vi "Solenoid Bank.vi"(0 "VISA session":refnum<visa-resource-name>="MW100", 1 "Semiphore":T1, 2 "Valve Bank":u16(ring) items=["A", "B", "C", "D"], 5 "Drain Valve":enum8{"OPEN", "CLOSE"}(ring)=enum."CLOSE", 7 "Output Valve":enum8{"CLOSE", "OPEN"}(ring)=enum."OPEN", 9 "Input Valve":enum8{"OPEN", "CLOSE"}(ring)=enum."CLOSE", 11 "Error In":errorcluster) -> (4 "dup VISA session":refnum<visa-resource-name>, 15 "Error Out":errorcluster)   [LabVIEW 2012]
uses:
  ChannelSettings.ctl
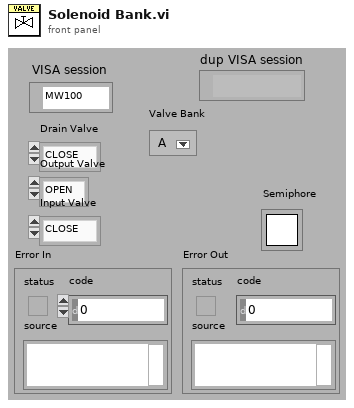
[diagram p1: front panel]
types:
  T1 = typedef "Semaphore RefNum" = refnum<k1>
  T2 = typedef "ChannelSettings.ctl" = u32
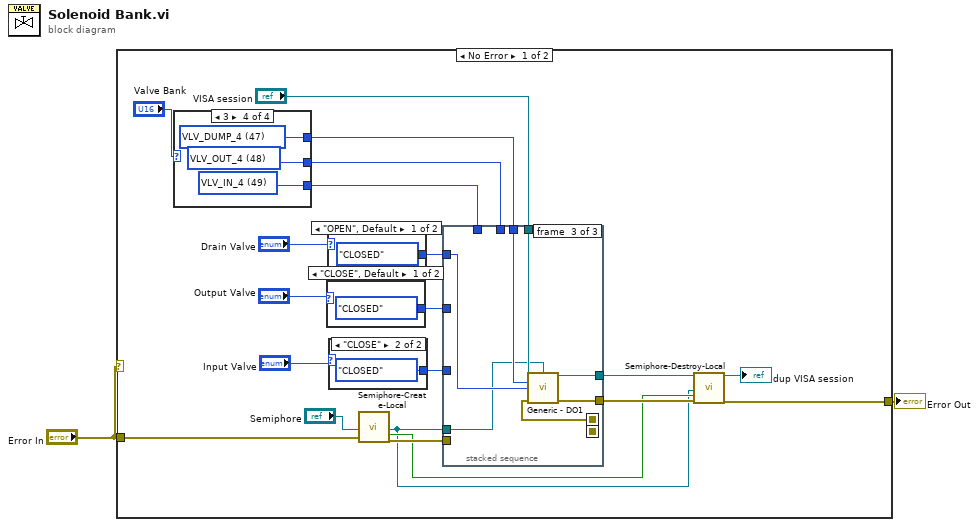
[diagram p0: block diagram]
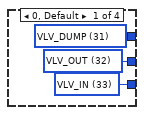
[diagram p2: hidden frame]
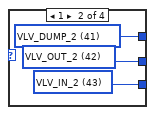
[diagram p3: hidden frame]
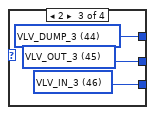
[diagram p4: hidden frame]
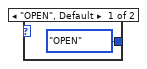
[diagram p5: hidden frame]
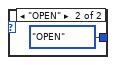
[diagram p6: hidden frame]
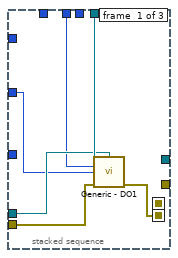
[diagram p7: hidden frame]
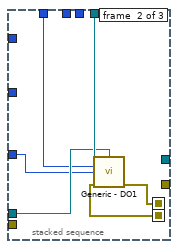
[diagram p8: hidden frame]
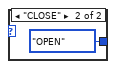
[diagram p9: hidden frame]
diagram:
  n1 = case shown="No Error" "Error In" {
    tunnel: "Error In" -> [w15 w59]
    tunnel: [w12 w59] -> w1
    frame No Error {
      n2 = case shown="3" "Valve Bank" {
        tunnel: [w24 w27 w30 w33] -> w17
        tunnel: [w23 w26 w29 w32] -> w5
        tunnel: [w22 w25 w28 w31] -> w4
        frame 0, Default {
          w22 = T2 33 items=["4-20_OUT", "Pres_HI1", "Pres_HI2", "Pres_LOW", "Pres_PIN", "HEATER_TOP", "HEATER_BOT", "T_Shell", "FLOWMETER", "WATT_SENSE", "WH_TICK", "Tc_1", "Tc_2", "Tc_3", "Tc_4", "Tc_5", "Tc_6", "Tc_down", "T_Shell_2", "T_Shell_3", "T_Shell_4", "RTD_IN", "RTD_OUT", "RTD_AMB", "INTF_TEMPFLO", "INTF_READY", "INTF_START", "INTF_STOP", "DRM_LOW", "DRM_HIGH", "PWR_MAIN", "VLV_DUMP", "VLV_OUT", "VLV_IN", "WATT_HOURS", "FLOW(SAMPLE)", "GALLONS", "FLOW(GPM)"] ("Channel_Enum")
          w23 = T2 32 items=["4-20_OUT", "Pres_HI1", "Pres_HI2", "Pres_LOW", "Pres_PIN", "HEATER_TOP", "HEATER_BOT", "T_Shell", "FLOWMETER", "WATT_SENSE", "WH_TICK", "Tc_1", "Tc_2", "Tc_3", "Tc_4", "Tc_5", "Tc_6", "Tc_down", "T_Shell_2", "T_Shell_3", "T_Shell_4", "RTD_IN", "RTD_OUT", "RTD_AMB", "INTF_TEMPFLO", "INTF_READY", "INTF_START", "INTF_STOP", "DRM_LOW", "DRM_HIGH", "PWR_MAIN", "VLV_DUMP", "VLV_OUT", "VLV_IN", "WATT_HOURS", "FLOW(SAMPLE)", "GALLONS", "FLOW(GPM)"] ("Channel_Enum")
          w24 = T2 31 items=["4-20_OUT", "Pres_HI1", "Pres_HI2", "Pres_LOW", "Pres_PIN", "HEATER_TOP", "HEATER_BOT", "T_Shell", "FLOWMETER", "WATT_SENSE", "WH_TICK", "Tc_1", "Tc_2", "Tc_3", "Tc_4", "Tc_5", "Tc_6", "Tc_down", "T_Shell_2", "T_Shell_3", "T_Shell_4", "RTD_IN", "RTD_OUT", "RTD_AMB", "INTF_TEMPFLO", "INTF_READY", "INTF_START", "INTF_STOP", "DRM_LOW", "DRM_HIGH", "PWR_MAIN", "VLV_DUMP", "VLV_OUT", "VLV_IN", "WATT_HOURS", "FLOW(SAMPLE)", "GALLONS", "FLOW(GPM)"] ("Channel_Enum")
        }
        frame 1 {
          w25 = T2 43 items=["4-20_OUT", "Pres_HI1", "Pres_HI2", "Pres_LOW", "Pres_PIN", "HEATER_TOP", "HEATER_BOT", "T_Shell", "FLOWMETER", "WATT_SENSE", "WH_TICK", "Tc_1", "Tc_2", "Tc_3", "Tc_4", "Tc_5", "Tc_6", "Tc_down", "T_Shell_2", "T_Shell_3", "T_Shell_4", "RTD_IN", "RTD_OUT", "RTD_AMB", "INTF_TEMPFLO", "INTF_READY", "INTF_START", "INTF_STOP", "DRM_LOW", "DRM_HIGH", "PWR_MAIN", "VLV_DUMP", "VLV_OUT", "VLV_IN", "WATT_HOURS", "FLOW(SAMPLE)", "GALLONS", "FLOW(GPM)", "FLOW_CALC_GAIN", "FLOW_CALC_OFFSET", "FLOW_CALC_THRESHOLD", "VLV_DUMP_2", "VLV_OUT_2", "VLV_IN_2", "VLV_DUMP_3", "VLV_OUT_3", "VLV_IN_3", "VLV_DUMP_4", "VLV_OUT_4", "VLV_IN_4"] ("Channel_Enum")
          w26 = T2 42 items=["4-20_OUT", "Pres_HI1", "Pres_HI2", "Pres_LOW", "Pres_PIN", "HEATER_TOP", "HEATER_BOT", "T_Shell", "FLOWMETER", "WATT_SENSE", "WH_TICK", "Tc_1", "Tc_2", "Tc_3", "Tc_4", "Tc_5", "Tc_6", "Tc_down", "T_Shell_2", "T_Shell_3", "T_Shell_4", "RTD_IN", "RTD_OUT", "RTD_AMB", "INTF_TEMPFLO", "INTF_READY", "INTF_START", "INTF_STOP", "DRM_LOW", "DRM_HIGH", "PWR_MAIN", "VLV_DUMP", "VLV_OUT", "VLV_IN", "WATT_HOURS", "FLOW(SAMPLE)", "GALLONS", "FLOW(GPM)", "FLOW_CALC_GAIN", "FLOW_CALC_OFFSET", "FLOW_CALC_THRESHOLD", "VLV_DUMP_2", "VLV_OUT_2", "VLV_IN_2", "VLV_DUMP_3", "VLV_OUT_3", "VLV_IN_3", "VLV_DUMP_4", "VLV_OUT_4", "VLV_IN_4"] ("Channel_Enum")
          w27 = T2 41 items=["4-20_OUT", "Pres_HI1", "Pres_HI2", "Pres_LOW", "Pres_PIN", "HEATER_TOP", "HEATER_BOT", "T_Shell", "FLOWMETER", "WATT_SENSE", "WH_TICK", "Tc_1", "Tc_2", "Tc_3", "Tc_4", "Tc_5", "Tc_6", "Tc_down", "T_Shell_2", "T_Shell_3", "T_Shell_4", "RTD_IN", "RTD_OUT", "RTD_AMB", "INTF_TEMPFLO", "INTF_READY", "INTF_START", "INTF_STOP", "DRM_LOW", "DRM_HIGH", "PWR_MAIN", "VLV_DUMP", "VLV_OUT", "VLV_IN", "WATT_HOURS", "FLOW(SAMPLE)", "GALLONS", "FLOW(GPM)", "FLOW_CALC_GAIN", "FLOW_CALC_OFFSET", "FLOW_CALC_THRESHOLD", "VLV_DUMP_2", "VLV_OUT_2", "VLV_IN_2", "VLV_DUMP_3", "VLV_OUT_3", "VLV_IN_3", "VLV_DUMP_4", "VLV_OUT_4", "VLV_IN_4"] ("Channel_Enum")
        }
        frame 2 {
          w28 = T2 46 items=["4-20_OUT", "Pres_HI1", "Pres_HI2", "Pres_LOW", "Pres_PIN", "HEATER_TOP", "HEATER_BOT", "T_Shell", "FLOWMETER", "WATT_SENSE", "WH_TICK", "Tc_1", "Tc_2", "Tc_3", "Tc_4", "Tc_5", "Tc_6", "Tc_down", "T_Shell_2", "T_Shell_3", "T_Shell_4", "RTD_IN", "RTD_OUT", "RTD_AMB", "INTF_TEMPFLO", "INTF_READY", "INTF_START", "INTF_STOP", "DRM_LOW", "DRM_HIGH", "PWR_MAIN", "VLV_DUMP", "VLV_OUT", "VLV_IN", "WATT_HOURS", "FLOW(SAMPLE)", "GALLONS", "FLOW(GPM)", "FLOW_CALC_GAIN", "FLOW_CALC_OFFSET", "FLOW_CALC_THRESHOLD", "VLV_DUMP_2", "VLV_OUT_2", "VLV_IN_2", "VLV_DUMP_3", "VLV_OUT_3", "VLV_IN_3", "VLV_DUMP_4", "VLV_OUT_4", "VLV_IN_4"] ("Channel_Enum")
          w29 = T2 45 items=["4-20_OUT", "Pres_HI1", "Pres_HI2", "Pres_LOW", "Pres_PIN", "HEATER_TOP", "HEATER_BOT", "T_Shell", "FLOWMETER", "WATT_SENSE", "WH_TICK", "Tc_1", "Tc_2", "Tc_3", "Tc_4", "Tc_5", "Tc_6", "Tc_down", "T_Shell_2", "T_Shell_3", "T_Shell_4", "RTD_IN", "RTD_OUT", "RTD_AMB", "INTF_TEMPFLO", "INTF_READY", "INTF_START", "INTF_STOP", "DRM_LOW", "DRM_HIGH", "PWR_MAIN", "VLV_DUMP", "VLV_OUT", "VLV_IN", "WATT_HOURS", "FLOW(SAMPLE)", "GALLONS", "FLOW(GPM)", "FLOW_CALC_GAIN", "FLOW_CALC_OFFSET", "FLOW_CALC_THRESHOLD", "VLV_DUMP_2", "VLV_OUT_2", "VLV_IN_2", "VLV_DUMP_3", "VLV_OUT_3", "VLV_IN_3", "VLV_DUMP_4", "VLV_OUT_4", "VLV_IN_4"] ("Channel_Enum")
          w30 = T2 44 items=["4-20_OUT", "Pres_HI1", "Pres_HI2", "Pres_LOW", "Pres_PIN", "HEATER_TOP", "HEATER_BOT", "T_Shell", "FLOWMETER", "WATT_SENSE", "WH_TICK", "Tc_1", "Tc_2", "Tc_3", "Tc_4", "Tc_5", "Tc_6", "Tc_down", "T_Shell_2", "T_Shell_3", "T_Shell_4", "RTD_IN", "RTD_OUT", "RTD_AMB", "INTF_TEMPFLO", "INTF_READY", "INTF_START", "INTF_STOP", "DRM_LOW", "DRM_HIGH", "PWR_MAIN", "VLV_DUMP", "VLV_OUT", "VLV_IN", "WATT_HOURS", "FLOW(SAMPLE)", "GALLONS", "FLOW(GPM)", "FLOW_CALC_GAIN", "FLOW_CALC_OFFSET", "FLOW_CALC_THRESHOLD", "VLV_DUMP_2", "VLV_OUT_2", "VLV_IN_2", "VLV_DUMP_3", "VLV_OUT_3", "VLV_IN_3", "VLV_DUMP_4", "VLV_OUT_4", "VLV_IN_4"] ("Channel_Enum")
        }
        frame 3 {
          w31 = T2 49 items=["4-20_OUT", "Pres_HI1", "Pres_HI2", "Pres_LOW", "Pres_PIN", "HEATER_TOP", "HEATER_BOT", "T_Shell", "FLOWMETER", "WATT_SENSE", "WH_TICK", "Tc_1", "Tc_2", "Tc_3", "Tc_4", "Tc_5", "Tc_6", "Tc_down", "T_Shell_2", "T_Shell_3", "T_Shell_4", "RTD_IN", "RTD_OUT", "RTD_AMB", "INTF_TEMPFLO", "INTF_READY", "INTF_START", "INTF_STOP", "DRM_LOW", "DRM_HIGH", "PWR_MAIN", "VLV_DUMP", "VLV_OUT", "VLV_IN", "WATT_HOURS", "FLOW(SAMPLE)", "GALLONS", "FLOW(GPM)", "FLOW_CALC_GAIN", "FLOW_CALC_OFFSET", "FLOW_CALC_THRESHOLD", "VLV_DUMP_2", "VLV_OUT_2", "VLV_IN_2", "VLV_DUMP_3", "VLV_OUT_3", "VLV_IN_3", "VLV_DUMP_4", "VLV_OUT_4", "VLV_IN_4"] ("Channel_Enum")
          w32 = T2 48 items=["4-20_OUT", "Pres_HI1", "Pres_HI2", "Pres_LOW", "Pres_PIN", "HEATER_TOP", "HEATER_BOT", "T_Shell", "FLOWMETER", "WATT_SENSE", "WH_TICK", "Tc_1", "Tc_2", "Tc_3", "Tc_4", "Tc_5", "Tc_6", "Tc_down", "T_Shell_2", "T_Shell_3", "T_Shell_4", "RTD_IN", "RTD_OUT", "RTD_AMB", "INTF_TEMPFLO", "INTF_READY", "INTF_START", "INTF_STOP", "DRM_LOW", "DRM_HIGH", "PWR_MAIN", "VLV_DUMP", "VLV_OUT", "VLV_IN", "WATT_HOURS", "FLOW(SAMPLE)", "GALLONS", "FLOW(GPM)", "FLOW_CALC_GAIN", "FLOW_CALC_OFFSET", "FLOW_CALC_THRESHOLD", "VLV_DUMP_2", "VLV_OUT_2", "VLV_IN_2", "VLV_DUMP_3", "VLV_OUT_3", "VLV_IN_3", "VLV_DUMP_4", "VLV_OUT_4", "VLV_IN_4"] ("Channel_Enum")
          w33 = T2 47 items=["4-20_OUT", "Pres_HI1", "Pres_HI2", "Pres_LOW", "Pres_PIN", "HEATER_TOP", "HEATER_BOT", "T_Shell", "FLOWMETER", "WATT_SENSE", "WH_TICK", "Tc_1", "Tc_2", "Tc_3", "Tc_4", "Tc_5", "Tc_6", "Tc_down", "T_Shell_2", "T_Shell_3", "T_Shell_4", "RTD_IN", "RTD_OUT", "RTD_AMB", "INTF_TEMPFLO", "INTF_READY", "INTF_START", "INTF_STOP", "DRM_LOW", "DRM_HIGH", "PWR_MAIN", "VLV_DUMP", "VLV_OUT", "VLV_IN", "WATT_HOURS", "FLOW(SAMPLE)", "GALLONS", "FLOW(GPM)", "FLOW_CALC_GAIN", "FLOW_CALC_OFFSET", "FLOW_CALC_THRESHOLD", "VLV_DUMP_2", "VLV_OUT_2", "VLV_IN_2", "VLV_DUMP_3", "VLV_OUT_3", "VLV_IN_3", "VLV_DUMP_4", "VLV_OUT_4", "VLV_IN_4"] ("Channel_Enum")
        }
      }
      n3 = case shown="\"CLOSE\", Default" "Output Valve" {
        tunnel: [enum8{"CLOSED", "OPEN"}."CLOSED" ("Relay Status (0:CLOSED)") enum8{"CLOSED", "OPEN"}."OPEN" ("Relay Status (0:CLOSED)")] -> w8
        frame "CLOSE", Default {
        }
        frame "OPEN" {
        }
      }
      n4 = case shown="\"OPEN\", Default" "Drain Valve" {
        tunnel: [enum8{"CLOSED", "OPEN"}."CLOSED" ("Relay Status (0:CLOSED)") enum8{"CLOSED", "OPEN"}."OPEN" ("Relay Status (0:CLOSED)")] -> w19
        frame "OPEN", Default {
        }
        frame "CLOSE" {
        }
      }
      n5 = case shown="\"CLOSE\"" "Input Valve" {
        tunnel: [enum8{"CLOSED", "OPEN"}."OPEN" ("Relay Status (0:CLOSED)") enum8{"CLOSED", "OPEN"}."CLOSED" ("Relay Status (0:CLOSED)")] -> w6
        frame "OPEN", Default {
        }
        frame "CLOSE" {
        }
      }
      n6 = call "Semiphore-Create-Local.vi"("Semiphore"="Semiphore", "error in (no error)"=w15) -> ("semaphore"=w10:T1, "Local?"=w11:bool, "error out"=w14:errorcluster)  [unwired: 15 in]
      n7 = stacked-sequence {
        seq-local: [_ w44 _] -> [_ _ w51]
        seq-local: [w41 _ _] -> [_ w45 _]
        tunnel: [_ _ w56] -> w20
        tunnel: w19 -> [_ _ w55]
        tunnel: "VISA session" -> [w43 w49 w54]
        tunnel: w17 -> [_ _ w53]
        tunnel: w14 -> [w38 _ _]
        tunnel: [_ _ w50] -> w13
        tunnel: w10 -> [w42 w48 w52]
        tunnel: w8 -> [w40 _ _]
        tunnel: w6 -> [_ w47 _]
        tunnel: w5 -> [w39 _ _]
        tunnel: w4 -> [_ w46 _]
        frame #0 {
          n8 = call "Generic - DO1.vi"("VISA session"=w43, "Semiphore"=w42, "Channel_Enum"=w39, "Relay Status (0:CLOSED)"=w40, "Error In"=w38) -> ("error out"=w41:errorcluster)  [unwired: 9 in, 1 out]
        }
        frame #1 {
          n9 = call "Generic - DO1.vi"("VISA session"=w49, "Semiphore"=w48, "Channel_Enum"=w46, "Relay Status (0:CLOSED)"=w47, "Error In"=w45) -> ("error out"=w44:errorcluster)  [unwired: 9 in, 1 out]
        }
        frame #2 {
          n10 = call "Generic - DO1.vi"("VISA session"=w54, "Semiphore"=w52, "Channel_Enum"=w53, "Relay Status (0:CLOSED)"=w55, "Error In"=w51) -> ("dup VISA session"=w56:refnum<visa-resource-name>, "error out"=w50:errorcluster)  [unwired: 9 in]
        }
      }
      "dup VISA session" <- w20
      n11 = call "Semiphore-Destroy-Local.vi"("Semiphore"=w10, "Local?"=w11, "error in (no error)"=w13) -> ("error out"=w12:errorcluster)  [unwired: 16 in]
    }
    frame Error {
    }
  }
  "Error Out" <- w1
